vi "RT Main and Scoreboard_audio test.vi"() -> ()   [LabVIEW 2026]
uses:
  RT Image.ctl
  RT States.ctl
  Idle Pattern.ctl
  Score.ctl
  SideSelector.ctl
  RT Commands.ctl
  Game Settings.ctl
  2 Player Bitfile dynRef.ctl
  <vilib>/FPGAPlugInAG/cRIO-9047/niLvFpga_Open_cRIO-9047.vi
  <vilib>/rvi/interface/common/dynamic/niFpgaDynamicAddResources.vi
  <vilib>/FPGAPlugInAG/Dynamic/niLvFpga_Run_Dynamic.vi
  <vilib>/rvi/interface/common/niFpgaWaitOnOcc.vi
  <vilib>/Utility/error.llb/Error Cluster From Error Code.vi
  <vilib>/rvi/errors/niLvFpgaAdjustHostInterfaceError.vi
  <vilib>/FPGAPlugInAG/Dynamic/niLvFpga_Abort_Dynamic.vi
  <vilib>/FPGAPlugInAG/Dynamic/niLvFpga_Close_Dynamic.vi
  <vilib>/rvi/interface/nirviOpenFPGA/nirviOpenFPGA.xnode
  FPGA Bitfiles/speedofvight_FPGATarget_IdlePatternandSo_vDPccMaBPIg.lvbitx
  Idle Pattern and Sounds.vi
  <vilib>/rvi/interface/nirviMethod/nirviMethod.xnode
  <vilib>/rvi/interface/nirviReadWriteControl/nirviReadWriteControl.xnode
  <vilib>/rvi/interface/nirviCloseFPGA/nirviCloseFPGA.xnode
  FPGA Bitfiles/speedofvight_1Player.lvbitx
  FPGA Bitfiles/speedofvight_2Player.lvbitx
  FPGA Bitfiles/speedofvight_IdlePattern.lvbitx
  <vilib>/rvi/interface/Simulation/niFpgaSimulationCallBeginRW.vi
  NiFpgaLv.dll
  <vilib>/Utility/Data Type/NI_Data Type.lvlib
  <vilib>/rvi/errors/niLvFpgaMergeErrorWithErrorCode.vi
  <vilib>/FPGAPlugInAG/Dynamic/niLvFpga_ConfigureFifo_Dynamic.vi
  <vilib>/FPGAPlugInAG/Dynamic/niLvFpga_WriteFifo_Dynamic.vi
panel:
  out "appended path":path
  out "Array Size":i32
  in  "Audio ON":bool
  out "Empty Elements Remaining":u32
  out "audio data":i16[](array[numeric])
  out "Actual Depth":u32
  out "error out 3":errorcluster
  out "x-y*floor(x/y)":u32
  out "floor(x/y)":u32
  in  "Winner Display time, ms":u32=7000
  in  "2 Players":bool
  in  "Idle Pattern Cycle Time":u32=5000
  in  "abort":bool
  in  "End Idle":bool
  out "error out":errorcluster
  in  "Speed Threshold, ticks":u64=3000
  in  "Debounce Threshold, ticks":u64=5000
  in  "Game Time":u32=4
  in  "End Game":bool
  out "Score P1":u16 format="%03.0f"
  out "Score P2":u16 format="%03.0f"
  out "2D Picture":T1
  out "Time Remaining":u32 format="%03.0f"
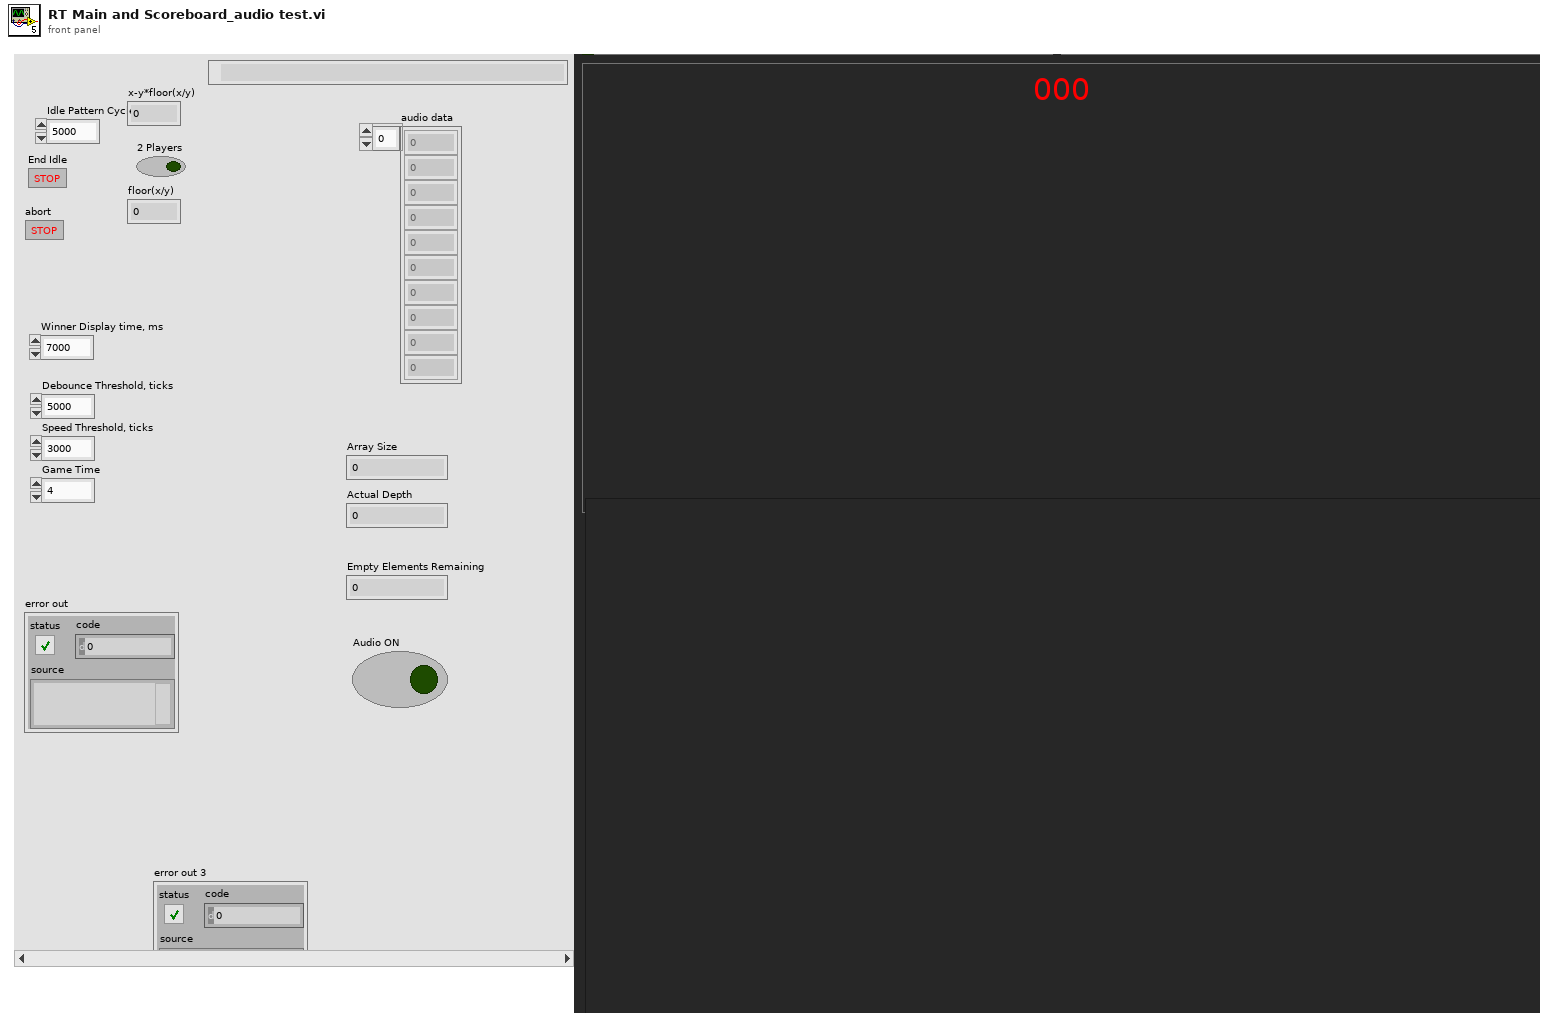
[diagram p1: front panel]
types:
  T1 = typedef "RT Image.ctl" = picture
  T2 = typedef "Score.ctl" = cluster{"Score P1":u16, "Score P2":u16, "Winner Selection":T3}
  T3 = typedef "SideSelector.ctl" = enum16{"P12", "P1", "P2"}
  T4 = cluster{"Debounce Threshold, ticks":u64, "Speed Threshold, ticks":u64, "Game Time":u32, "Idle Pattern Cycle Time, ms":u32, "Winner Display time, ms":u32, "Final Score":T2}
  T5 = typedef "Idle Pattern.ctl" = enum16{"Expanding Circle", "Plasma", "Radar Sweep", "Matrix Rain", "Campfire", "Diagonal Scan", "LV40"}
  T6 = typedef "RT States.ctl" = enum16{"Idle", "Configuring", "1Player", "2Player", "Display Winner"}
  T7 = typedef "RT Commands.ctl" = enum16{"<null>", "End Idle", "Reset", "Commit Settings", "Commit Host Settings"}
  T8 = typedef "2 Player Bitfile dynRef.ctl" = refnum<k20>
  T9 = typedef "Game Settings.ctl" = cluster{"Speed Threshold, ticks":u64, "Game Time":u32, "2 Players":bool}
  T10 = cluster{"Score P1":u16, "Score P2":u16, "Winner Selection":T3}
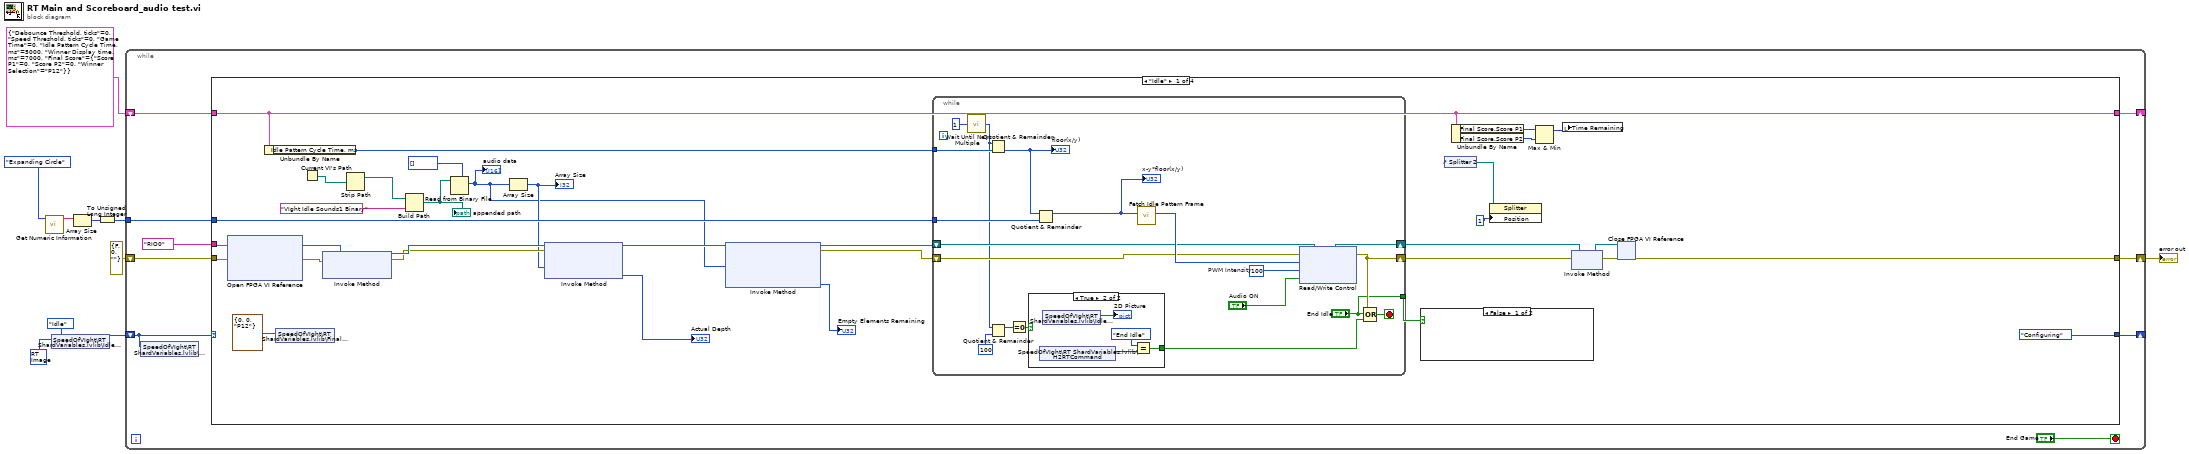
[diagram p0: block diagram]
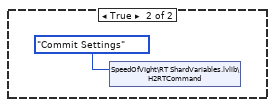
[diagram p2: hidden frame]
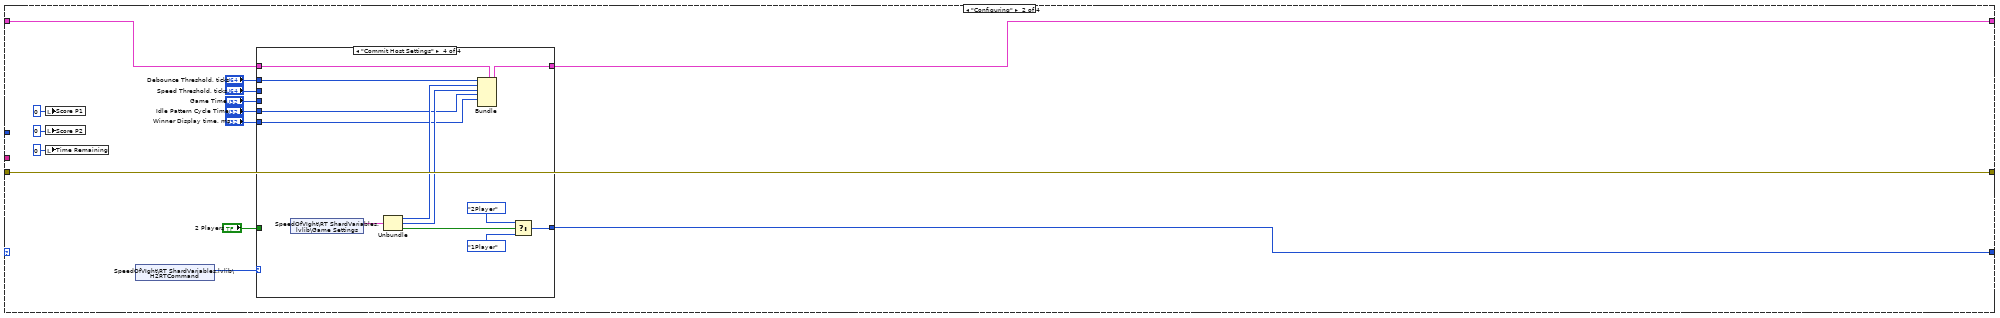
[diagram p4: hidden frame]
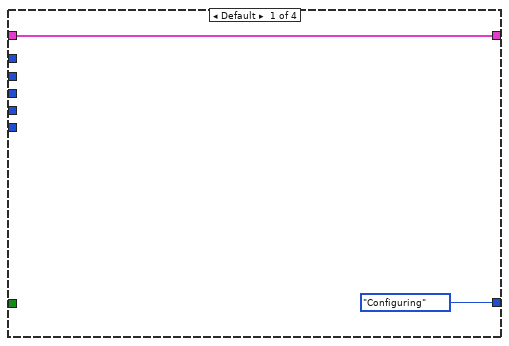
[diagram p5: hidden frame]
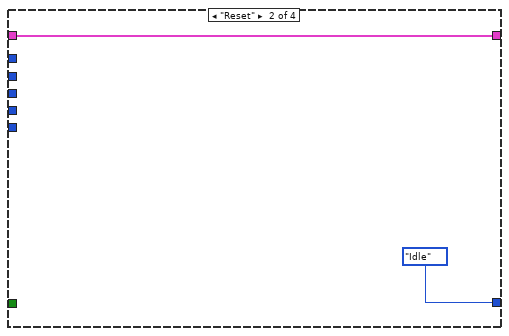
[diagram p6: hidden frame]
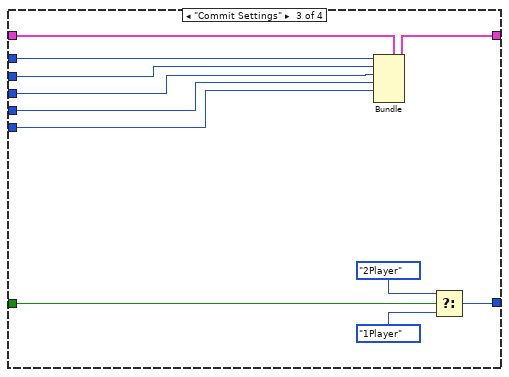
[diagram p7: hidden frame]
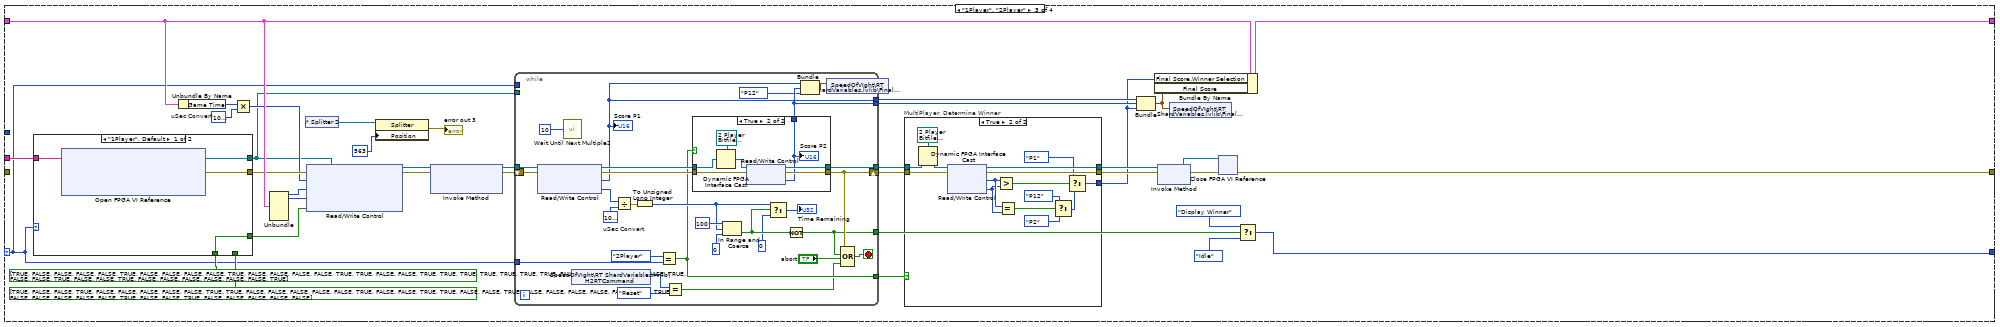
[diagram p8: hidden frame]
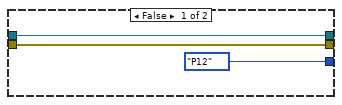
[diagram p9: hidden frame]
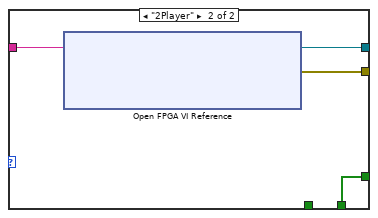
[diagram p10: hidden frame]
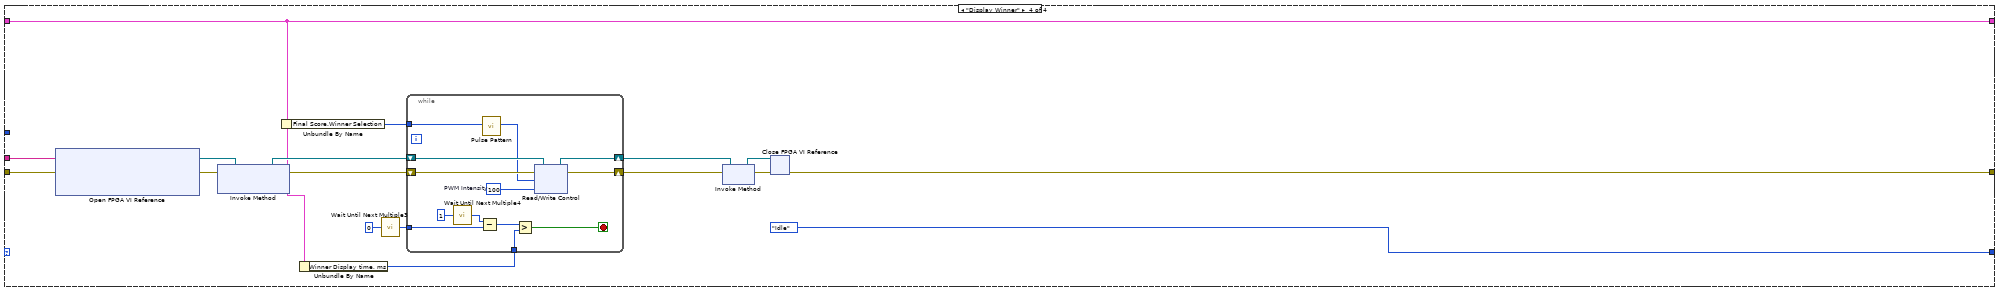
[diagram p12: hidden frame]
diagram:
  n1 = call <vilib>:"Get Numeric Information.vi"("variant"=Idle_Pattern."Expanding Circle" ("Effect")) -> ("enum names"=w7:string[])  [unwired: 7 in, 3 out]
  n2 = shared-variable "SpeedOfVIght\\RT ShardVariables.lvlib\\Idle Image"(T1 data[5B] ("Idle Image")) -> ()  [unwired: 1 in, 1 out]
  n3 = Array Size(array=w7) -> (size(s)=w6:i32)
  n4 = To Unsigned Long Integer(number=w6) -> (unsigned 32bit integer=w2:u32)
  n5 = while {
    shift-right: [w14] -> _
    shift-left: RT_States."Idle" ("Enum") -> [w11]
    tunnel: w2 -> [w17]
    shift-right: [w16] -> w5
    shift-left: errorcluster {"status"=FALSE, "code"=0, "source"=""} ("error out") -> [w15]
    shift-right: [w12] -> _
    shift-left: T4 {"Debounce Threshold, ticks"=0, "Speed Threshold, ticks"=0, "Game Time"=0, "Idle Pattern Cycle Time, ms"=5000, "Winner Display time, ms"=7000, "Final Score"={"Score P1"=0, "Score P2"=0, "Winner Selection"=enum."P12"}} ("cluster") -> [w13]
    stop <- "End Game" stop-if-true
    n6 = shared-variable "SpeedOfVIght\\RT ShardVariables.lvlib\\RT2HState"(w11) -> ()  [unwired: 1 in, 1 out]
    n7 = case shown="\"Idle\"" w11 {
      selector: w11 -> [_ _ w123 _]
      tunnel: tag "RIO0" ("resource name") -> [w22 _ w146 w231]
      tunnel: w17 -> [w52 _ _ _]
      tunnel: [w47 w90 w140 w226] -> w16
      tunnel: w15 -> [w21 w90 _ w225]
      tunnel: [RT_States."Configuring" ("Enum") w87 w133 RT_States."Idle" ("Enum")] -> w14
      tunnel: w13 -> [w41 w89 w154 w219]
      tunnel: [w41 w88 w134 w219] -> w12
      frame "Idle" {
        n8 = xnode "Open FPGA VI Reference"("error in"=w21, "resource name"=w22) -> ("FPGA VI Reference Out"=w20:refnum<k20>, "error out"=w19:errorcluster)
        n9 = Unbundle By Name(w41) -> ("Idle Pattern Cycle Time, ms"=w45:u32)
        n10 = shared-variable "SpeedOfVIght\\RT ShardVariables.lvlib\\Final Score"(T2 {"Score P1"=0, "Score P2"=0, "Winner Selection"=enum."P12"} ("Final Score")) -> ()  [unwired: 1 in, 1 out]
        n11 = Current VI's Path() -> (path=w34:path)
        n12 = xnode "Invoke Method"("FPGA VI Reference In"=w20, "error in"=w19) -> ("FPGA VI Reference Out"=w36:refnum<k20>, "error out"=w35:errorcluster)  [unwired: 1 in]
        n13 = Strip Path(path=w34) -> (stripped path=w33:path)  [unwired: 1 out]
        n14 = Build Path(base path=w33, name or relative path="VIght Idle Sounds1 Binary") -> (appended path=w31:path)
        "appended path" <- w31
        n15 = Read from Binary File(5:i16[] [], 11:w31) -> (2:w26:i16[])  [unwired: 4 in, 3 out]
        "audio data" <- w26
        n16 = Array Size(array=w26) -> (size(s)=w29:i32)
        "Array Size" <- w29
        n17 = xnode "Invoke Method"("FPGA VI Reference In"=w36, "error in"=w35, "Requested Depth"=w29) -> ("FPGA VI Reference Out"=w27:refnum<k20>, "Actual Depth"=→"Actual Depth":u32)  [unwired: 1 out]
        n18 = xnode "Invoke Method"("FPGA VI Reference In"=w27, "Data"=w26) -> ("FPGA VI Reference Out"=w24:refnum<k20>, "error out"=w23:errorcluster, "Empty Elements Remaining"=→"Empty Elements Remaining":u32)  [unwired: 2 in]
        n19 = while {
          shift-right: [w64] -> w49
          shift-left: w23 -> [w70]
          shift-right: [w68] -> w48
          shift-left: w24 -> [w69]
          tunnel: w52 -> [w62]
          tunnel: w45 -> [w63]
          tunnel: ["End Idle"] -> w44
          stop <- w66 stop-if-true
          w71 = u16 100  # PWM Intensity
          n20 = call "Wait Until Next Multiple"("Count(mSec)"=u32 1 ("Count(Ticks)")) -> ("Tick Count(mSec)"=w57:u32)
          n21 = Quotient & Remainder(x=w57, y=w63) -> (floor(x/y)=w61:u32)  [unwired: 1 out]
          "floor(x/y)" <- w61
          n22 = Quotient & Remainder(x=w57, y=u32 100) -> (x-y*floor(x/y)=w55:u32)  [unwired: 1 out]
          n23 = Equal To 0?(x=w55) -> (x = 0?=w58:bool)
          n24 = case shown="True" w58 {
            tunnel: [_ w75] -> w65
            frame False {
            }
            frame True {
              n25 = shared-variable "SpeedOfVIght\\RT ShardVariables.lvlib\\H2RTCommand"() -> (w74:T7)  [unwired: 1 in, 1 out]
              n26 = shared-variable "SpeedOfVIght\\RT ShardVariables.lvlib\\Idle Image"() -> (→"2D Picture":T1)  [unwired: 1 in, 1 out]
              n27 = Equal?(x=RT_Commands."End Idle", y=w74) -> (x = y?=w75:bool)
            }
          }
          n28 = Quotient & Remainder(x=w61, y=w62) -> (x-y*floor(x/y)=w60:u32)  [unwired: 1 out]
          "x-y*floor(x/y)" <- w60
          n29 = call "Fetch Idle Pattern Frame.vi"("Effect"=w60) -> ("Array"=w72:u16[])  [unwired: 10 in]
          n30 = xnode "Read/Write Control"("FPGA VI Reference In"=w69, "error in"=w70, "x"=w72, "Period"=w71, "Turn On Audio"="Audio ON") -> ("FPGA VI Reference Out"=w68:refnum<k20>, "error out"=w64:errorcluster)
          n31 = Compound Arithmetic op=OR(w64, "End Idle", w65) -> (w66:bool)
        }
        n32 = case shown="False" w44 {
          frame False {
          }
          frame True {
            n33 = shared-variable "SpeedOfVIght\\RT ShardVariables.lvlib\\H2RTCommand"(RT_Commands."Commit Settings" ("H2RTCommand")) -> ()  [unwired: 1 in, 1 out]
          }
        }
        n34 = control-ref of="Splitter 2"() -> (w42:refnum<vi>)
        n35 = Unbundle By Name(w41) -> ("Final Score.Score P1"=w40:u16, "Final Score.Score P2"=w39:u16)
        n36 = property class="Splitter"(reference=w42, "Position"=1 ("Splitter Position")) -> ()  [unwired: 1 in, 2 out]
        n37 = Max & Min(x=w40, y=w39) -> (max(x,y)=w38:u16)  [unwired: 1 out]
        n38 = local write "Time Remaining"(w38) -> ()
        n39 = xnode "Invoke Method"("FPGA VI Reference In"=w48, "error in"=w49) -> ("FPGA VI Reference Out"=w51:refnum<k20>, "error out"=w50:errorcluster)
        n40 = xnode "Close FPGA VI Reference"("FPGA VI Reference In"=w51, "error in"=w50) -> ("error out"=w47:errorcluster)
      }
      frame "Configuring" {
        n41 = local write "Score P1"(u16 0 ("Score P1")) -> ()
        n42 = local write "Score P2"(u16 0 ("Score P2")) -> ()
        n43 = local write "Time Remaining"(u32 0 ("Time Remaining")) -> ()
        n44 = shared-variable "SpeedOfVIght\\RT ShardVariables.lvlib\\H2RTCommand"() -> (w83:T7)  [unwired: 1 in, 1 out]
        n45 = case shown="\"Commit Host Settings\"" w83 {
          tunnel: w89 -> [w91 w94 w103 w115]
          tunnel: [w91 w94 w102 w114] -> w88
          tunnel: [RT_States."Configuring" ("Enum") RT_States."Idle" ("Enum") w101 w113] -> w87
          tunnel: "Winner Display time, ms" -> [_ _ w95 w106]
          tunnel: "Idle Pattern Cycle Time" -> [_ _ w96 w107]
          tunnel: "Speed Threshold, ticks" -> [_ _ w100 _]
          tunnel: "Debounce Threshold, ticks" -> [_ _ w99 w112]
          tunnel: "Game Time" -> [_ _ w98 _]
          tunnel: "2 Players" -> [_ _ w97 _]
          frame Default {
          }
          frame "Reset" {
          }
          frame "Commit Settings" {
            n46 = Bundle(cluster=w103, "Debounce Threshold, ticks"=w99, "Speed Threshold, ticks"=w100, "Game Time"=w98, "Idle Pattern Cycle Time, ms"=w96, "Winner Display time, ms"=w95) -> (w102:T4)  [unwired: 1 in]
            n47 = Select(t=RT_States."2Player" ("Enum"), s=w97, f=RT_States."1Player" ("Enum")) -> (s? t:f=w101:T6)
          }
          frame "Commit Host Settings" {
            n48 = shared-variable "SpeedOfVIght\\RT ShardVariables.lvlib\\Game Settings"() -> (w111:T9)  [unwired: 1 in, 1 out]
            n49 = Unbundle(w111) -> ("Speed Threshold, ticks"=w110:u64, "Game Time"=w108:u32, "2 Players"=w109:bool)
            n50 = Bundle(cluster=w115, "Debounce Threshold, ticks"=w112, "Speed Threshold, ticks"=w110, "Game Time"=w108, "Idle Pattern Cycle Time, ms"=w107, "Winner Display time, ms"=w106) -> (w114:T4)  [unwired: 1 in]
            n51 = Select(t=RT_States."2Player" ("Enum"), s=w109, f=RT_States."1Player" ("Enum")) -> (s? t:f=w113:T6)
          }
        }
      }
      frame "1Player", "2Player" {
        w153 = u32 1000000  # uSec Convert
        n52 = case shown="\"1Player\", Default" w123 {
          tunnel: [w176 w180] -> w150
          tunnel: [w175 w179] -> w122
          tunnel: w146 -> [w174 w178]
          tunnel: [w173 w177] -> w121
          tunnel: bool[] [TRUE, FALSE, FALSE, TRUE, FALSE, FALSE, FALSE, FALSE, FALSE, TRUE, TRUE, FALSE, FALSE, FALSE, FALSE, FALSE, TRUE, FALSE, FALSE, TRUE, TRUE, FALSE, FALSE, TRUE, FALSE, FALSE, FALSE, FALSE, FALSE, TRUE, TRUE, FALSE, FALSE, FALSE, FALSE, FALSE, TRUE, FALSE, FALSE, TRUE, FALSE, FALSE, FALSE, FALSE, FALSE] ("appended array") -> [_ w177]
          tunnel: bool[] [TRUE, FALSE, FALSE, FALSE, FALSE, TRUE, FALSE, FALSE, FALSE, FALSE, TRUE, FALSE, FALSE, FALSE, FALSE, TRUE, TRUE, FALSE, FALSE, TRUE, TRUE, TRUE, TRUE, TRUE, TRUE, TRUE, FALSE, FALSE, TRUE, FALSE, FALSE, TRUE, FALSE, FALSE, TRUE, FALSE, FALSE, TRUE, FALSE, FALSE, FALSE, FALSE, FALSE, FALSE, TRUE] ("appended array") -> [w173 _]
          frame "1Player", Default {
            n53 = xnode "Open FPGA VI Reference"("resource name"=w174) -> ("FPGA VI Reference Out"=w175:refnum<k20>, "error out"=w176:errorcluster)  [unwired: 1 in]
          }
          frame "2Player" {
            n54 = xnode "Open FPGA VI Reference"("resource name"=w178) -> ("FPGA VI Reference Out"=w179:refnum<k20>, "error out"=w180:errorcluster)  [unwired: 1 in]
          }
        }
        n55 = Unbundle By Name(w154) -> ("Game Time"=w143:u32)
        n56 = Multiply(x=w143, y=w153) -> (x*y=w147:u32)
        n57 = Unbundle(w154) -> ("Debounce Threshold, ticks"=w145:u64, "Speed Threshold, ticks"=w144:u64)  [unwired: 4 out]
        n58 = control-ref of="Splitter 2"() -> (w120:refnum<vi>)
        n59 = xnode "Read/Write Control"("FPGA VI Reference In"=w122, "error in"=w150, "Game Time, uS"=w147, "Debounce Threshold, ticks"=w145, "Speed Threshold, ticks"=w144, "Starting Lights"=w121) -> ("FPGA VI Reference Out"=w148:refnum<k20>, "error out"=w149:errorcluster)
        n60 = property class="Splitter"(reference=w120, "Position"=563 ("Splitter Position")) -> (error out=→"error out 3":errorcluster)  [unwired: 1 in, 1 out]
        n61 = xnode "Invoke Method"("FPGA VI Reference In"=w148, "error in"=w149) -> ("FPGA VI Reference Out"=w152:refnum<k20>, "error out"=w151:errorcluster)  [unwired: 1 in]
        n62 = while {
          tunnel: w152 -> [w209]
          shift-right: [w202] -> w137
          shift-left: w151 -> [w208]
          tunnel: w123 -> [w200]
          tunnel: [w196] -> w138
          tunnel: [w189] -> w131
          tunnel: [w188] -> w139
          tunnel: [w184] -> w127
          tunnel: [w183] -> w126
          tunnel: w123 -> [_]
          tunnel: w122 -> [_]
          stop <- w203 stop-if-true
          w206 = u32 1000000  # uSec Convert
          n63 = xnode "Read/Write Control"("FPGA VI Reference In"=w209, "error in"=w208) -> ("FPGA VI Reference Out"=w201:refnum<k20>, "error out"=w204:errorcluster, "Score P1"=w184:u16, "Time Remaining"=w193:u32)
          "Score P1" <- w184
          n64 = call "Wait Until Next Multiple2"("Count(mSec)"=u32 10 ("Count(Ticks)")) -> ()  [unwired: 1 out]
          n65 = shared-variable "SpeedOfVIght\\RT ShardVariables.lvlib\\H2RTCommand"() -> (w185:T7)  [unwired: 1 in, 1 out]
          n66 = Divide(x=w193, y=w206) -> (x/y=w207:dbl)
          n67 = To Unsigned Long Integer(number=w207) -> (unsigned 32bit integer=w190:u32)
          n68 = Equal?(x=RT_States."2Player", y=w200) -> (x = y?=w188:bool)
          n69 = Equal?(x=w185, y=RT_Commands."Reset") -> (x = y?=w186:bool)
          n70 = case shown="True" w188 {
            tunnel: w204 -> [w211 w218]
            tunnel: [w211 w217] -> w202
            tunnel: w201 -> [w210 w215]
            tunnel: [w210 w213] -> w196
            tunnel: [_ w212] -> w183
            frame False {
            }
            frame True {
              n71 = Dynamic FPGA Interface Cast(Session In=T8 refnum ("FPGA Interface"), Type=w215) -> (Session Out=w214:T8)
              n72 = xnode "Read/Write Control"("FPGA VI Reference In"=w214, "error in"=w218) -> ("FPGA VI Reference Out"=w213:T8, "error out"=w217:errorcluster, "Score P2"=w212:u16)
              "Score P2" <- w212
            }
          }
          n73 = In Range and Coerce(upper limit=u32 100, x=w190, lower limit=u32 0 ("y")) -> (In Range?=w194:bool)  [unwired: 1 out]
          n74 = Select(t=w190, s=w194, f=u32 0 ("y")) -> (s? t:f=→"Time Remaining":u32)
          n75 = Not(x=w194) -> (.not. x?=w189:bool)
          n76 = Bundle("Score P1"=w184, "Score P2"=w183, "Winner Selection"=SideSelector."P12") -> (w181:T10)  [unwired: 1 in]
          n77 = shared-variable "SpeedOfVIght\\RT ShardVariables.lvlib\\Final Score"(w181) -> ()  [unwired: 1 in, 1 out]
          n78 = Compound Arithmetic op=OR(w202, w189, "abort", w186) -> (w203:bool)
        }
        n79 = case "MultiPlayer, Determine Winner" shown="True" w139 {
          tunnel: w138 -> [w156 w168]
          tunnel: w137 -> [w157 w172]
          tunnel: [w157 w171] -> w136
          tunnel: [w156 w170] -> w135
          tunnel: [SideSelector."P12" ("Winner Selection") w163] -> w124
          frame False {
          }
          frame True {
            n80 = Dynamic FPGA Interface Cast(Session In=T8 refnum ("FPGA Interface"), Type=w168) -> (Session Out=w169:T8)
            n81 = xnode "Read/Write Control"("FPGA VI Reference In"=w169, "error in"=w172) -> ("FPGA VI Reference Out"=w170:T8, "error out"=w171:errorcluster, "Score P1"=w166:u16, "Score P2"=w162:u16)
            n82 = Greater?(x=w166, y=w162) -> (0:w167:bool)
            n83 = Equal?(x=w166, y=w162) -> (x = y?=w165:bool)
            n84 = Select(t=SideSelector."P12" ("Winner Selection"), s=w165, f=SideSelector."P2" ("Winner Selection")) -> (s? t:f=w159:T3)
            n85 = Select(t=SideSelector."P1" ("Winner Selection"), s=w167, f=w159) -> (s? t:f=w163:T3)
          }
        }
        n86 = Bundle("Score P1"=w127, "Score P2"=w126, "Winner Selection"=w124) -> (w125:T10)  [unwired: 1 in]
        n87 = Bundle By Name(cluster=w154, "Final Score.Winner Selection"=w124, "Final Score"=w125) -> (w134:T4)
        n88 = xnode "Invoke Method"("FPGA VI Reference In"=w135, "error in"=w136) -> ("FPGA VI Reference Out"=w142:refnum<k20>, "error out"=w141:errorcluster)
        n89 = shared-variable "SpeedOfVIght\\RT ShardVariables.lvlib\\Final Score"(w125) -> ()  [unwired: 1 in, 1 out]
        n90 = xnode "Close FPGA VI Reference"("FPGA VI Reference In"=w142, "error in"=w141) -> ("error out"=w140:errorcluster)
        n91 = Select(t=RT_States."Display Winner" ("Enum"), s=w131, f=RT_States."Idle" ("Enum")) -> (s? t:f=w133:T6)
      }
      frame "Display Winner" {
        n92 = xnode "Open FPGA VI Reference"("error in"=w225, "resource name"=w231) -> ("FPGA VI Reference Out"=w233:refnum<k20>, "error out"=w235:errorcluster)
        n93 = xnode "Invoke Method"("FPGA VI Reference In"=w233, "error in"=w235) -> ("FPGA VI Reference Out"=w232:refnum<k20>, "error out"=w234:errorcluster)  [unwired: 1 in]
        n94 = Unbundle By Name(w219) -> ("Final Score.Winner Selection"=w223:T3)
        n95 = Unbundle By Name(w219) -> ("Winner Display time, ms"=w220:u32)
        n96 = call "Wait Until Next Multiple3"("Count(mSec)"=u32 0 ("Count(Ticks)")) -> ("Tick Count(mSec)"=w221:u32)
        n97 = while {
          shift-right: [w248] -> w228
          shift-left: w234 -> [w246]
          shift-right: [w244] -> w227
          shift-left: w232 -> [w245]
          tunnel: w223 -> [w243]
          tunnel: w221 -> [w239]
          tunnel: w220 -> [w237]
          stop <- w236 stop-if-true
          w247 = u16 100  # PWM Intensity
          n98 = call "Wait Until Next Multiple4"("Count(mSec)"=u32 1 ("Count(Ticks)")) -> ("Tick Count(mSec)"=w240:u32)
          n99 = Subtract(x=w240, y=w239) -> (x-y=w238:u32)
          n100 = call "Pulse Pattern.vi"("Selector"=w243) -> ("Array"=w242:u16[])  [unwired: 10 in]
          n101 = Greater?(x=w238, y=w237) -> (0:w236:bool)
          n102 = xnode "Read/Write Control"("FPGA VI Reference In"=w245, "error in"=w246, "x"=w242, "Period"=w247) -> ("FPGA VI Reference Out"=w244:refnum<k20>, "error out"=w248:errorcluster)
        }
        n103 = xnode "Invoke Method"("FPGA VI Reference In"=w227, "error in"=w228) -> ("FPGA VI Reference Out"=w230:refnum<k20>, "error out"=w229:errorcluster)
        n104 = xnode "Close FPGA VI Reference"("FPGA VI Reference In"=w230, "error in"=w229) -> ("error out"=w226:errorcluster)
      }
    }
  }
  "error out" <- w5
